vi "GlobalSetGetPixelOfRoi.vi"() -> ()   [LabVIEW 2013]
panel:
  in  "Scanspeed":dbl
  in  "CyclesZ":dbl
  in  "TNum":dbl
  in  "TDelta":dbl
  in  "Points":dbl
  in  "CyclesY":dbl
  in  "Y length":dbl
  in  "Y Start":dbl
  in  "X length":dbl
  in  "X Start":dbl
  in  "Stepsize X":dbl
  in  "Stepsize Y":dbl
  in  "Stepsize Z":dbl
  in  "Stack length":dbl
  in  "Stack Start":dbl
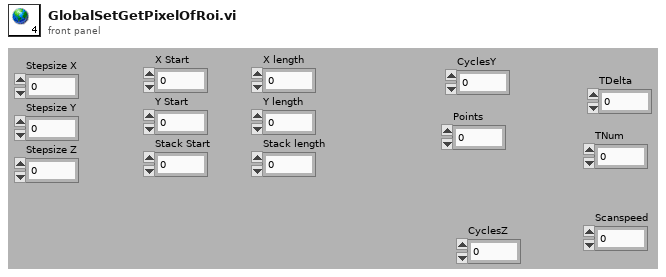
[diagram p1: front panel]
diagram:
